vi "Data_Aquisition_cRIO5_slim.vi"() -> ()   [LabVIEW 2016]
uses:
  <vilib>/Platform/TimedLoop/XDataNode/timing_clust.ctl
  <vilib>/Platform/TimedLoop/XDataNode/nitl_modes.ctl
  <vilib>/Platform/TimedLoop/XDataNode/wakeup.ctl
  <vilib>/Utility/file.llb/Write Delimited Spreadsheet (string).vi
  <vilib>/Platform/TimedLoop/XDataNode/loadnilvce.vi
  <vilib>/Utility/file.llb/Write Delimited Spreadsheet (DBL).vi
  <vilib>/Platform/TimedLoop/XDataNode/XDataNode.xnode
  <vilib>/Platform/TimedLoop/XDataNode/XDNodeRunTimeDep.lvlib
panel:
  in  "Mod 1":string[][](array[string])=[["M1DO4", "M1DO3"], ["NH4", "HCO3"]]
  in  "Mod 3":string[][](array[string])=[["M3AI0", "M3AI1", "M3AI2", "M3AI3"], ["pH", "DO", "Air", "N2"]]
  out "Data":dbl[][](array[numeric])=[[9.0, 6.0, 2018.0, 8492636.0, 0.0, 0.012268418868999998, 0.004043026478000001, 0.004586713565, 0.004174119744]]
  out "Headers":string[][](array[string])=[["Month", "Day", "Year", "Time", "M1DO4", "M3AI0", "M3AI1", "M3AI2", "M3AI3"], ["Month", "Day", "Year", "Time", "NH4", "pH", "DO", "Air", "N2"]]
  out "Time":string="084926.36"
  out "Date":string="09062018"
  in  "Buffer Size":i32=6
  out "Saving?":bool=TRUE
  out "new file path (Not A Path if cancelled)":path=path "u:/_09052018_102926.csv"
  in  "File Name:":string
  out "error out":errorcluster
  out "iter number":i32=134
  in  "stop":bool
  in  "error in":errorcluster
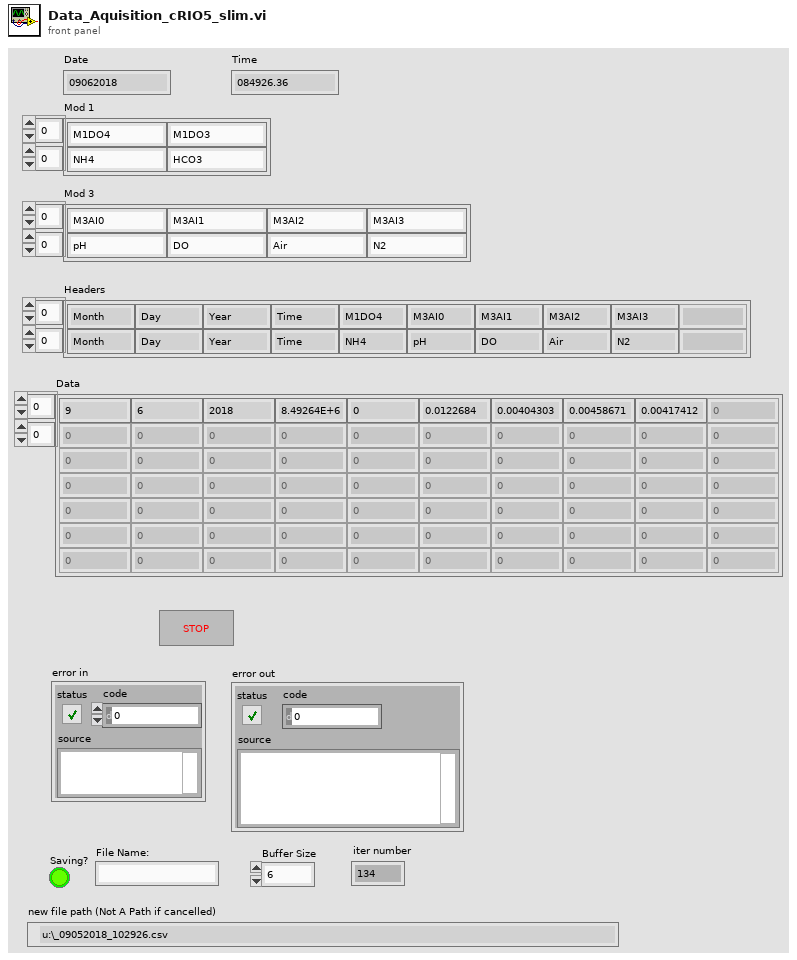
[diagram p1: front panel]
types:
  T1 = typedef "XDNodeRunTimeDep.lvlib/timing_clust.ctl" = cluster{"Expected End [f-1]":u64, "Actual End [f-1]":u64, "Finished Late? [f-1]":bool, "Expected End [i-1]":u64, "Actual End [i-1]":u64, "Finished Late? [i-1]":bool, "Expected Start [i]":u64, "Actual Start [i]":u64, "Expected Start [f]":u64, "Actual Start [f]":u64, "Source Name":string, "Structure Name":string, "Period":i64, "Deadline":i64, "Offset":i64, "Start":i64, "Priority":i32, "Timeout":i32, "Mode":T2, "Wakeup Reason":T3, "Error":errorcluster, "Source Type":string, "Secondary Source Type":string, "Global End Time":u64, "Global Start Time":u64, "Frame Duration":u64, "Iteration Duration":u64, "Assigned CPU":i32, "I/O Scan Engine Mode":u32}
  T2 = typedef "XDNodeRunTimeDep.lvlib/nitl_modes.ctl" = enum32{"No Change", "Process missed periods, maintain original phase", "Discard missed periods, maintain original phase", "Process missed periods, ignore original phase", "Discard missed periods, ignore original phase"}
  T3 = typedef "XDNodeRunTimeDep.lvlib/wakeup.ctl" = enum32{"Normal", "Aborted", "Asynchronous wakeup", "Timing source error", "Timed loop error", "Timeout"}
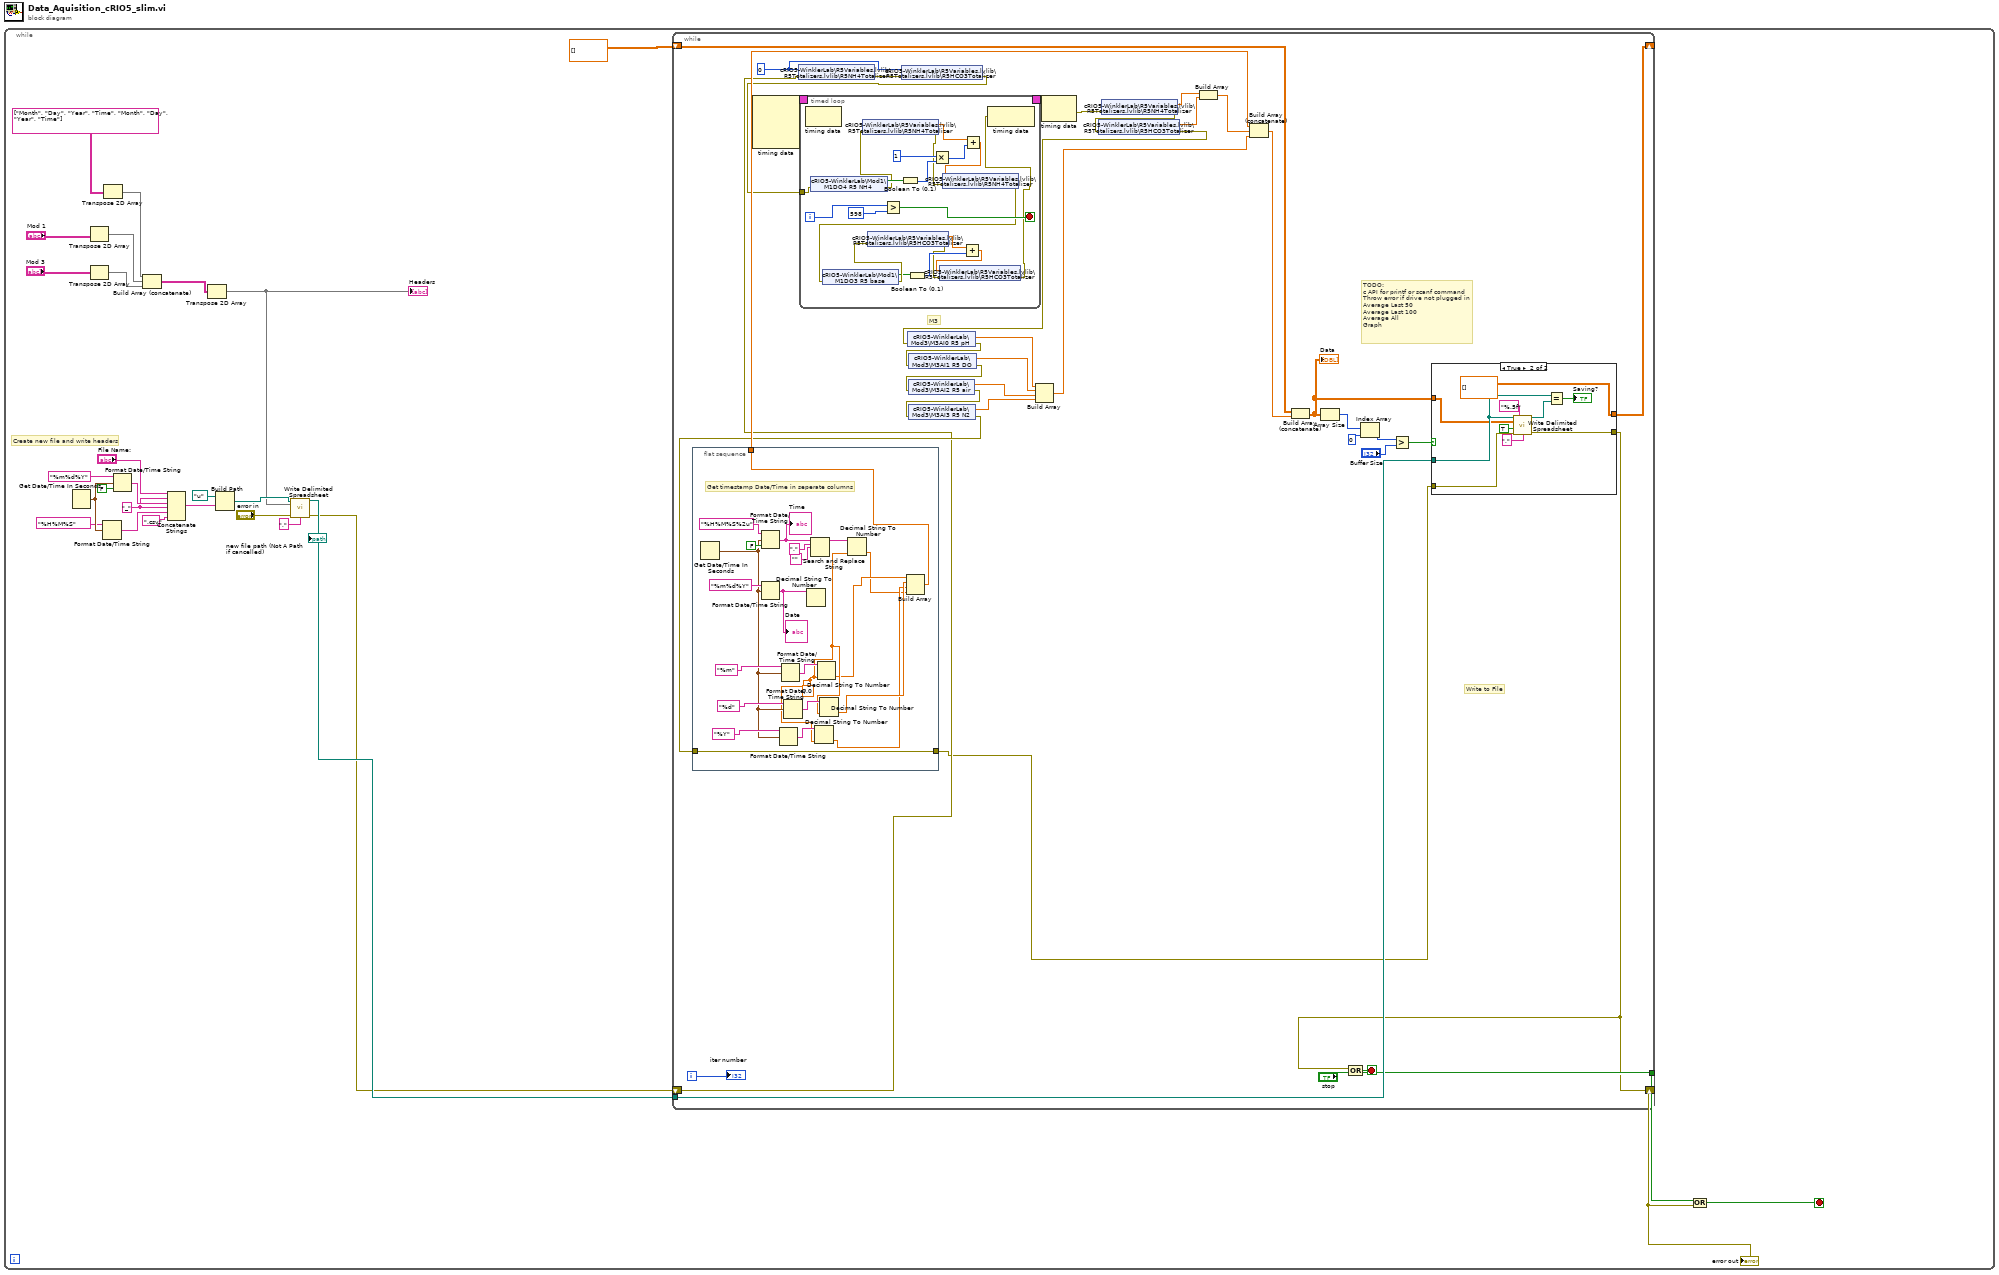
[diagram p0: block diagram]
diagram:
  n1 = while {
    stop <- w3 stop-if-true
    w16 = "_" ("string")
    # "Create new file and write headers"
    n2 = Get Date/Time In Seconds() -> (seconds since 1Jan1904=w21:timestamp)
    n3 = Transpose 2D Array(2D array="Mod 1") -> (transposed array=w5:string[][])
    n4 = Transpose 2D Array(2D array="Mod 3") -> (transposed array=w6:string[][])
    n5 = Format Date/Time String(time format string (%c)="%H%M%S", seconds (now)=w21) -> (date/time string=w15:string)  [unwired: 1 in]
    n6 = Transpose 2D Array(2D array=string[][] [["Month", "Day", "Year", "Time"], ["Month", "Day", "Year", "Time"]]) -> (transposed array=w9:string[][])
    n7 = Format Date/Time String(time format string (%c)="%m%d%Y", seconds (now)=w21, UTC format=FALSE) -> (date/time string=w17:string)
    n8 = Build Array (concatenate)(w9, w5, w6) -> (w11:string[][])
    n9 = Concatenate Strings("File Name:", w16, w17, w16, w15, ".csv" ("string")) -> (w14:string)
    n10 = Transpose 2D Array(2D array=w11) -> (transposed array=w8:string[][])
    "Headers" <- w8
    n11 = Build Path(base path=path "u:/" ("Save to:"), name or relative path=w14) -> (appended path=w24:path)
    n12 = call-poly <vilib>:"Write Delimited Spreadsheet.vi"("file path (dialog if empty)"=w24, "2D data"=w8, "error in (no error)"="error in", "delimiter (\\t)"="," ("delimiter (\\t)")) -> ("new file path (Not A Path if cancelled)"=w28:path, "error out"=w27:errorcluster)  [unwired: 10 in]
    "new file path (Not A Path if cancelled)" <- w28
    n13 = while {
      tunnel: w28 -> [w58]
      shift-right: [w55] -> _
      shift-left: dbl[][] [] -> [w63]
      shift-right: [w29] -> w1
      shift-left: w27 -> [w39]
      tunnel: ["stop"] -> w2
      i -> [w64]
      stop <- w65 stop-if-true
      w36 = 0
      # "M3"
      # "TODO: \nc API for printf or scanf command\nThrow error if drive not plugged in\nAverage Last 50\nAverage Last 100\nAverage All\nGraph"
      # "Write to File"
      n14 = flat-sequence {
        tunnel: [w67] -> w54
        tunnel: [w66] -> w30
        tunnel: w40 -> [w66]
        frame #0 {
          w72 = 0.0
          # "Get timestamp Date/Time in seperate columns"
          n15 = Get Date/Time In Seconds() -> (seconds since 1Jan1904=w73:timestamp)
          n16 = Format Date/Time String(time format string (%c)="%H%M%S%2u", seconds (now)=w73, UTC format=FALSE) -> (date/time string=w84:string)
          "Time" <- w84
          n17 = Format Date/Time String(time format string (%c)="%m%d%Y", seconds (now)=w73) -> (date/time string=w81:string)  [unwired: 1 in]
          "Date" <- w81
          n18 = Format Date/Time String(time format string (%c)="%Y", seconds (now)=w73) -> (date/time string=w74:string)  [unwired: 1 in]
          n19 = Format Date/Time String(time format string (%c)="%m", seconds (now)=w73) -> (date/time string=w78:string)  [unwired: 1 in]
          n20 = Format Date/Time String(time format string (%c)="%d", seconds (now)=w73) -> (date/time string=w76:string)  [unwired: 1 in]
          n21 = Decimal String To Number(string=w81) -> ()  [unwired: 2 in, 2 out]
          n22 = Search and Replace String(input string=w84, search string=".", replace string="") -> (result string=w83:string)  [unwired: 5 in, 3 out]
          n23 = Decimal String To Number(string=w74, default (0L)=w72) -> (number=w69:dbl)  [unwired: 1 in, 1 out]
          n24 = Decimal String To Number(string=w78, default (0L)=w72) -> (number=w71:dbl)  [unwired: 1 in, 1 out]
          n25 = Decimal String To Number(string=w76, default (0L)=w72) -> (number=w70:dbl)  [unwired: 1 in, 1 out]
          n26 = Decimal String To Number(string=w83, default (0L)=w72) -> (number=w68:dbl)  [unwired: 1 in, 1 out]
          n27 = Build Array(w71, w70, w69, w68) -> (w67:dbl[])
        }
      }
      n28 = node-c288() -> (w43:T1)  [unwired: 4 in]
      n29 = shared-variable "cRIO5-WinklerLab\\R5Variables.lvlib\\R5Totalizers.lvlib\\R5NH4Totalizer"(w36, error in=w39) -> (error out=w38:errorcluster)
      n30 = shared-variable "cRIO5-WinklerLab\\R5Variables.lvlib\\R5Totalizers.lvlib\\R5HCO3Totalizer"(w36, error in=w38) -> (error out=w37:errorcluster)
      n31 = timed-loop {
        timing: w43 -> [_]
        timing-out: [_] -> w42
        tunnel: w37 -> [w101]
        i -> [w96]
        stop <- w98 stop-if-true
        n32 = node-c288() -> ()  [unwired: 1 in, 1 out]
        n33 = shared-variable "cRIO5-WinklerLab\\Mod1\\M1DO4 R5 NH4"(error in=w101) -> (w102:bool, error out=w100:errorcluster)
        n34 = shared-variable "cRIO5-WinklerLab\\R5Variables.lvlib\\R5Totalizers.lvlib\\R5NH4Totalizer"(error in=w100) -> (w106:dbl, error out=w99:errorcluster)
        n35 = Greater?(x=w96, y=598) -> (0:w98:bool)
        n36 = Boolean To (0,1)(Boolean=w102) -> (0, 1=w104:i16)
        n37 = Multiply(x=1, y=w104) -> (x*y=w105:i32)
        n38 = Add(x=w106, y=w105) -> (x+y=w107:dbl)
        n39 = shared-variable "cRIO5-WinklerLab\\R5Variables.lvlib\\R5Totalizers.lvlib\\R5NH4Totalizer"(w107, error in=w99) -> (error out=w93:errorcluster)
        n40 = shared-variable "cRIO5-WinklerLab\\Mod1\\M1DO3 R5 base"(error in=w93) -> (w90:bool, error out=w95:errorcluster)
        n41 = shared-variable "cRIO5-WinklerLab\\R5Variables.lvlib\\R5Totalizers.lvlib\\R5HCO3Totalizer"(error in=w95) -> (w92:dbl, error out=w89:errorcluster)
        n42 = Boolean To (0,1)(Boolean=w90) -> (0, 1=w91:i16)
        n43 = Add(x=w92, y=w91) -> (x+y=w88:dbl)
        n44 = shared-variable "cRIO5-WinklerLab\\R5Variables.lvlib\\R5Totalizers.lvlib\\R5HCO3Totalizer"(w88, error in=w89) -> (error out=w94:errorcluster)
        n45 = node-c288(w94) -> ()  [unwired: 1 out]
      }
      n46 = node-c288(w42) -> (w41:errorcluster)
      n47 = shared-variable "cRIO5-WinklerLab\\R5Variables.lvlib\\R5Totalizers.lvlib\\R5NH4Totalizer"(error in=w41) -> (w34:dbl, error out=w31:errorcluster)
      n48 = shared-variable "cRIO5-WinklerLab\\R5Variables.lvlib\\R5Totalizers.lvlib\\R5HCO3Totalizer"(error in=w31) -> (w33:dbl, error out=w32:errorcluster)
      n49 = shared-variable "cRIO5-WinklerLab\\Mod3\\M3AI0 R5 pH"(error in=w32) -> (w52:dbl, error out=w53:errorcluster)
      n50 = shared-variable "cRIO5-WinklerLab\\Mod3\\M3AI1 R5 DO"(error in=w53) -> (w51:dbl, error out=w48:errorcluster)
      n51 = shared-variable "cRIO5-WinklerLab\\Mod3\\M3AI2 R5 air"(error in=w48) -> (w46:dbl, error out=w47:errorcluster)
      n52 = shared-variable "cRIO5-WinklerLab\\Mod3\\M3AI3 R5 N2"(error in=w47) -> (w45:dbl, error out=w40:errorcluster)
      n53 = Build Array(w52, w51, w46, w45) -> (w44:dbl[])
      n54 = Build Array(w34, w33) -> (w35:dbl[])
      n55 = Build Array (concatenate)(w54, w35, w44) -> (w49:dbl[])
      n56 = Build Array (concatenate)(w63, w49) -> (w50:dbl[][])
      "Data" <- w50
      n57 = Array Size(array=w50) -> (size(s)=w62:i32[])
      n58 = Index Array(array=w62, index=0) -> (element=w60:i32)
      n59 = Greater?(x=w60, y="Buffer Size") -> (0:w59:bool)
      n60 = case shown="True" w59 {
        tunnel: w50 -> [w116 w117]
        tunnel: w58 -> [_ w124]
        tunnel: [w116 dbl[][] []] -> w55
        tunnel: [w115 w123] -> w29
        tunnel: w30 -> [w115 w118]
        frame False {
        }
        frame True {
          n61 = call-poly <vilib>:"Write Delimited Spreadsheet.vi"("file path (dialog if empty)"=w124, "format (%.3f)"="%.5f", "2D data"=w117, "append to file? (new file:F)"=TRUE, "error in (no error)"=w118, "delimiter (\\t)"="," ("delimiter (\\t)")) -> ("new file path (Not A Path if cancelled)"=w125:path, "error out"=w123:errorcluster)  [unwired: 8 in]
          n62 = Equal?(x=w124, y=w125) -> (x = y?=→"Saving?":bool)
        }
      }
      n63 = Compound Arithmetic op=OR(w29, "stop") -> (w65:bool)
      "iter number" <- w64
    }
    "error out" <- w1
    n64 = Or(x=w2, y=w1) -> (x .or. y?=w3:bool)
  }
